vi "ErrorHandlerGFV4Redtide.vi"(7 "ErrorHandlerEnum":T1, 8 "error in (no error)":errorcluster, 9 "Acquiring Engine":refnum<user-event>, 10 "Measurement Queue":refnum<queue>, 11 "Stop Instrument Engine":refnum<user-event>) -> (0 "error out":errorcluster)   [LabVIEW 2013]
doc: "Use this template to build a VI to use as a subVI."
uses:
  ErrorHandleEnum4redtide.ctl
  Instrument Module Typedefs/AbsorptionStateEnum.ctl
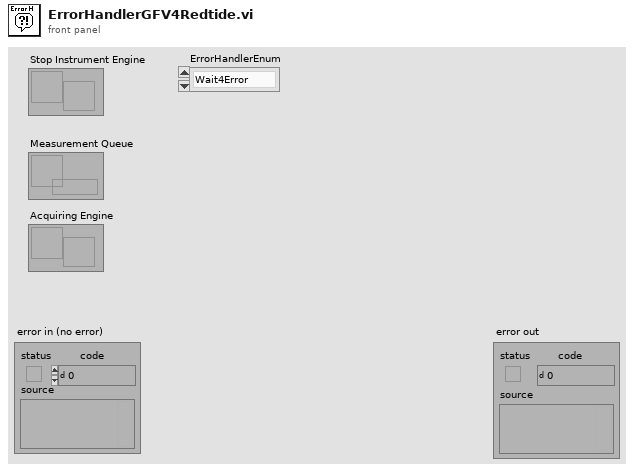
[diagram p1: front panel]
types:
  T1 = typedef "ErrorHandleEnum4redtide.ctl" = enum16{"Wait4Error", "Init"}
  T2 = typedef "AbsorptionStateEnum.ctl" = enum16{"RecieveMeasurement", "Stop Measurement Engine"}
  T3 = cluster{"Wavelength (nm)":dbl[], "Wavelength (nm)":dbl[]}
  T4 = cluster{"AbsMeas":T2, cluster{"Wavelength (nm)":dbl[], "Wavelength (nm)":dbl[]}}
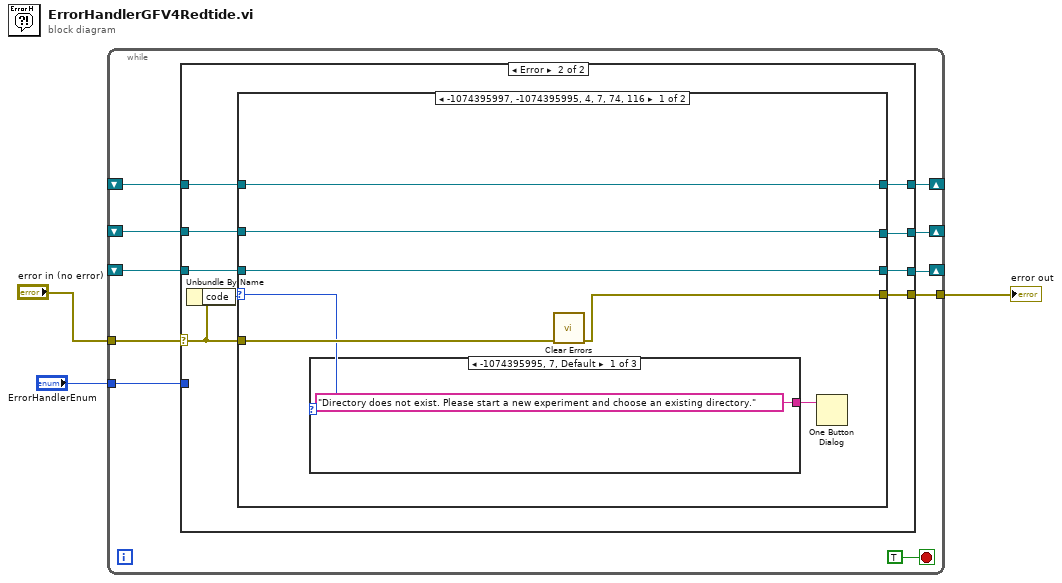
[diagram p0: block diagram]
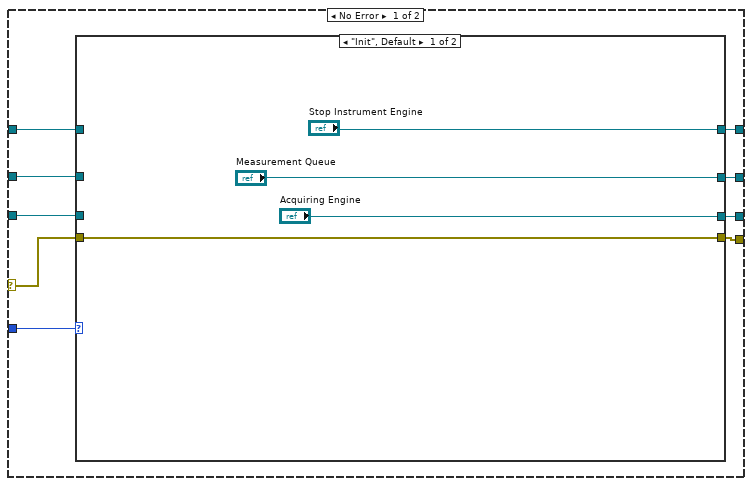
[diagram p2: hidden frame]
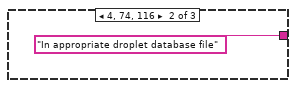
[diagram p4: hidden frame]
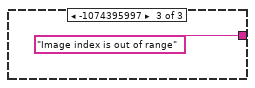
[diagram p5: hidden frame]
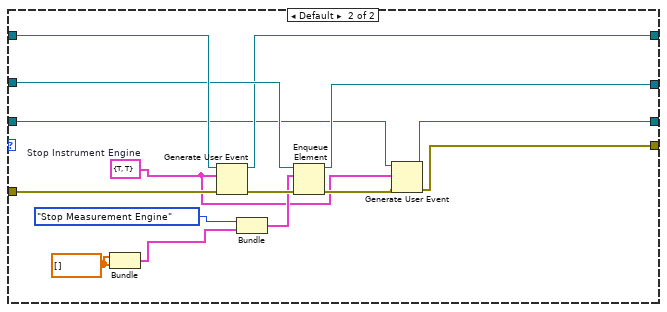
[diagram p6: hidden frame]
diagram:
  n1 = while {
    tunnel: "ErrorHandlerEnum" -> [w12]
    tunnel: "error in (no error)" -> [w8]
    shift-right: [w11] -> _
    shift-left: _ -> [w7]
    shift-right: [w10] -> _
    shift-left: _ -> [w6]
    shift-right: [w9] -> _
    shift-left: _ -> [w5]
    tunnel: [w4] -> w2
    stop <- TRUE stop-if-true
    n2 = case shown="Error" w8 {
      selector: w8 -> [w17 w34]
      tunnel: w12 -> [w22 _]
      tunnel: [w21 w31] -> w11
      tunnel: [w20 w37] -> w10
      tunnel: [w19 w35] -> w9
      tunnel: w7 -> [w16 w39]
      tunnel: w6 -> [w15 w38]
      tunnel: w5 -> [w14 w36]
      tunnel: [w18 w32] -> w4
      frame No Error {
        n3 = case shown="\"Init\", Default" w22 {
          tunnel: ["Stop Instrument Engine" w30] -> w21
          tunnel: ["Measurement Queue" w29] -> w20
          tunnel: ["Acquiring Engine" w28] -> w19
          tunnel: [w26 w27] -> w18
          tunnel: w17 -> [w26 w27]
          tunnel: w16 -> [_ w30]
          tunnel: w15 -> [_ w29]
          tunnel: w14 -> [_ w28]
          frame "Init", Default {
          }
          frame "Wait4Error" {
          }
        }
      }
      frame Error {
        n4 = Unbundle By Name(w34) -> ("code"=w33:i32)
        n5 = case shown="-1074395997, -1074395995, 4, 7, 74, 116" w33 {
          selector: w33 -> [w40 _]
          tunnel: w39 -> [w46 w64]
          tunnel: w38 -> [w45 w63]
          tunnel: [w45 w62] -> w37
          tunnel: w36 -> [w44 w53]
          tunnel: [w44 w50] -> w35
          tunnel: w34 -> [w43 w55]
          tunnel: [w42 w51] -> w32
          tunnel: [w46 w60] -> w31
          frame -1074395997, -1074395995, 4, 7, 74, 116 {
            n6 = case shown="-1074395995, 7, Default" w40 {
              tunnel: ["Directory does not exist. Please start a new experiment and choose an existing directory." ("message") "In appropriate droplet database file" ("message") "Image index is out of range" ("message")] -> w41
              frame -1074395995, 7, Default {
              }
              frame 4, 74, 116 {
              }
              frame -1074395997 {
              }
            }
            n7 = call <vilib>:"Clear Errors.vi"("error in (no error)"=w43) -> ("error out"=w42:errorcluster)  [unwired: 6 in]
            n8 = One Button Dialog(message=w41) -> ()  [unwired: 1 in, 1 out]
          }
          frame Default {
            w58 = dbl[] [] ("Wavelength (nm)")
            w52 = cluster{"stop":bool, "stop 2":bool} {"stop"=TRUE, "stop 2"=TRUE}  # Stop Instrument Engine
            n9 = Bundle("Wavelength (nm)"=w58, "Wavelength (nm)"=w58) -> (w57:T3)  [unwired: 1 in]
            n10 = Generate User Event(user event=w64, event data cluster=w52, error in=w55) -> (user event out=w60:refnum<user-event>, error out=w61:errorcluster)  [unwired: 1 in]
            n11 = Bundle("AbsMeas"=AbsorptionStateEnum."Stop Measurement Engine", w57) -> (w56:T4)  [unwired: 1 in]
            n12 = Enqueue Element(queue=w63, element=w56, error in (no error)=w61) -> (queue out=w62:refnum<queue>, error out=w54:errorcluster)  [unwired: 1 in, 1 out]
            n13 = Generate User Event(user event=w53, event data cluster=w52, error in=w54) -> (user event out=w50:refnum<user-event>, error out=w51:errorcluster)  [unwired: 1 in]
          }
        }
      }
    }
  }
  "error out" <- w2
